vi "MSEncoder SubVI WfmCodeGen_AmpScan.vi"(6 "AuxPulses":ext[](array[numeric]), 8 "AuxAmp":ext[](array[numeric]), 9 "Amp":ext[](array[numeric]), 10 "Scan time":ext, 11 "MSEncoder in":refnum<class "MSEncoder.lvclass">) -> (1 "Amp2":ext, 2 "WfmCode":u64[](array[numeric]))   [LabVIEW 2018, in "MSEncoder.lvclass"]
uses:
  MSEncoder.lvclass
  MSEncoder.lvclass/MSEncoder.ctl
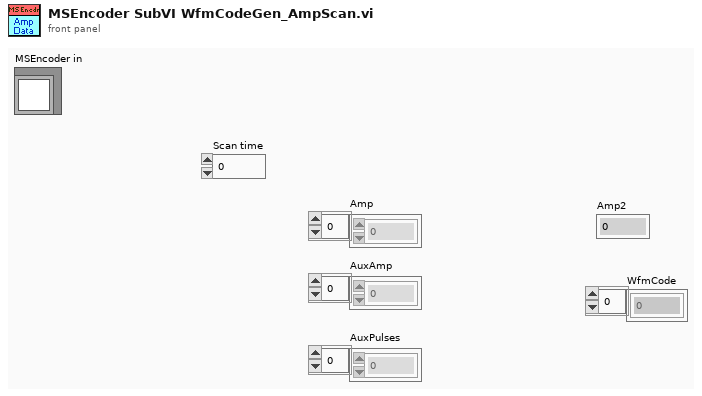
[diagram p1: front panel]
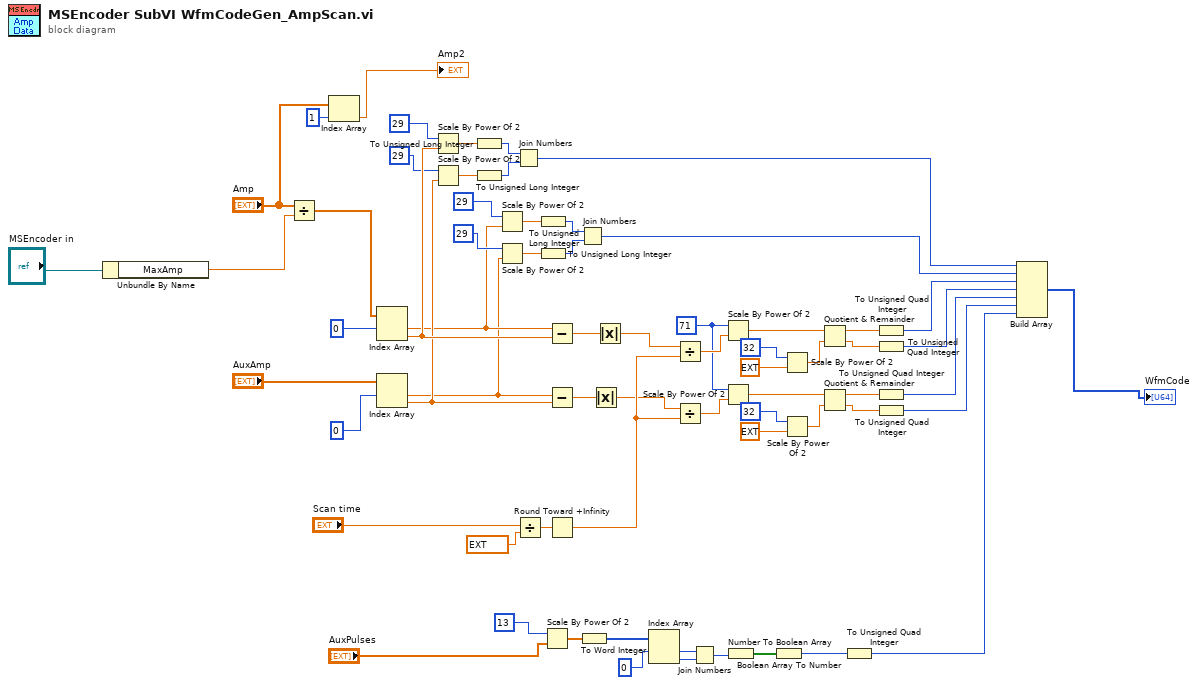
[diagram p0: block diagram]
diagram:
  w55 = i16 71 ("n")
  n1 = Unbundle By Name("MSEncoder in") -> ("MaxAmp"=w58:dbl)
  n2 = Divide(x="Amp", y=w58) -> (x/y=w52:ext[])
  n3 = Index Array(array="Amp", index=1) -> (element=→"Amp2":ext)
  n4 = Index Array(array=w52, index #1=0 ("index")) -> (element #1=w9:ext, element #2=w22:ext)  [unwired: 1 in]
  n5 = Index Array(array="AuxAmp", index #1=0 ("index")) -> (element #1=w8:ext, element #2=w19:ext)  [unwired: 1 in]
  n6 = Scale By Power Of 2(n=i16 29, x=w22) -> (x*2^n=w51:ext)
  n7 = Scale By Power Of 2(n=i16 29, x=w19) -> (x*2^n=w21:ext)
  n8 = To Unsigned Long Integer(number=w51) -> (unsigned 32bit integer=w18:u32)
  n9 = To Unsigned Long Integer(number=w21) -> (unsigned 32bit integer=w17:u32)
  n10 = Scale By Power Of 2(n=i16 29, x=w9) -> (x*2^n=w11:ext)
  n11 = Scale By Power Of 2(n=i16 29, x=w8) -> (x*2^n=w12:ext)
  n12 = Join Numbers(hi=w18, lo=w17) -> ((hi.lo)=w16:u64)
  n13 = Divide(x="Scan time", y=ext 2.5e-08) -> (x/y=w62:ext)
  n14 = To Unsigned Long Integer(number=w11) -> (unsigned 32bit integer=w14:u32)
  n15 = To Unsigned Long Integer(number=w12) -> (unsigned 32bit integer=w15:u32)
  n16 = Scale By Power Of 2(n=i16 13, x="AuxPulses") -> (x*2^n=w32:ext[])
  n17 = Subtract(x=w9, y=w22) -> (x-y=w5:ext)
  n18 = Subtract(x=w8, y=w19) -> (x-y=w66:ext)
  n19 = Round Toward +Infinity(x=w62) -> (ceil(x): smallest int >= x=w57:ext)
  n20 = Join Numbers(hi=w14, lo=w15) -> ((hi.lo)=w7:u64)
  n21 = To Word Integer(number=w32) -> (16bit integer=w31:i16[])
  n22 = Absolute Value(x=w66) -> (abs(x)=w4:ext)
  n23 = Absolute Value(x=w5) -> (abs(x)=w6:ext)
  n24 = Index Array(array=w31, index #1=0 ("index")) -> (element #1=w29:i16, element #2=w28:i16)  [unwired: 1 in]
  n25 = Divide(x=w6, y=w57) -> (x/y=w56:ext)
  n26 = Divide(x=w4, y=w57) -> (x/y=w54:ext)
  n27 = Join Numbers(hi=w29, lo=w28) -> ((hi.lo)=w27:u32)
  n28 = Scale By Power Of 2(n=w55, x=w56) -> (x*2^n=w47:ext)
  n29 = Scale By Power Of 2(n=w55, x=w54) -> (x*2^n=w43:ext)
  n30 = Number To Boolean Array(number=w27) -> (Boolean array=w26:bool[])
  n31 = Boolean Array To Number(Boolean array=w26) -> (number=w25:u32)
  n32 = Scale By Power Of 2(n=i16 32, x=ext 1.0) -> (x*2^n=w48:ext)
  n33 = Scale By Power Of 2(n=i16 32, x=ext 1.0) -> (x*2^n=w46:ext)
  n34 = Quotient & Remainder(x=w47, y=w48) -> (x-y*floor(x/y)=w42:ext, floor(x/y)=w40:ext)
  n35 = Quotient & Remainder(x=w43, y=w46) -> (x-y*floor(x/y)=w38:ext, floor(x/y)=w36:ext)
  n36 = To Unsigned Quad Integer(1:w25) -> (0:w24:u64)
  n37 = To Unsigned Quad Integer(1:w42) -> (0:w41:u64)
  n38 = To Unsigned Quad Integer(1:w40) -> (0:w39:u64)
  n39 = To Unsigned Quad Integer(1:w38) -> (0:w37:u64)
  n40 = To Unsigned Quad Integer(1:w36) -> (0:w35:u64)
  n41 = Build Array(w16, w7, w41, w39, w37, w35, w24) -> (→"WfmCode":u64[])
